vi "SectionA04_Week3_Stus.vi"() -> ()   [LabVIEW 2013]
uses:
  <vilib>/Platform/NI_3dgraph.lvlib
panel:
  in  "Bits":dbl(knob) scale=0.0..10.0
  in  "3D Surface":refnum<k7>(container)
  out "2^Bits":dbl
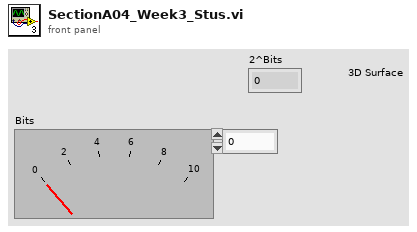
[diagram p1: front panel]
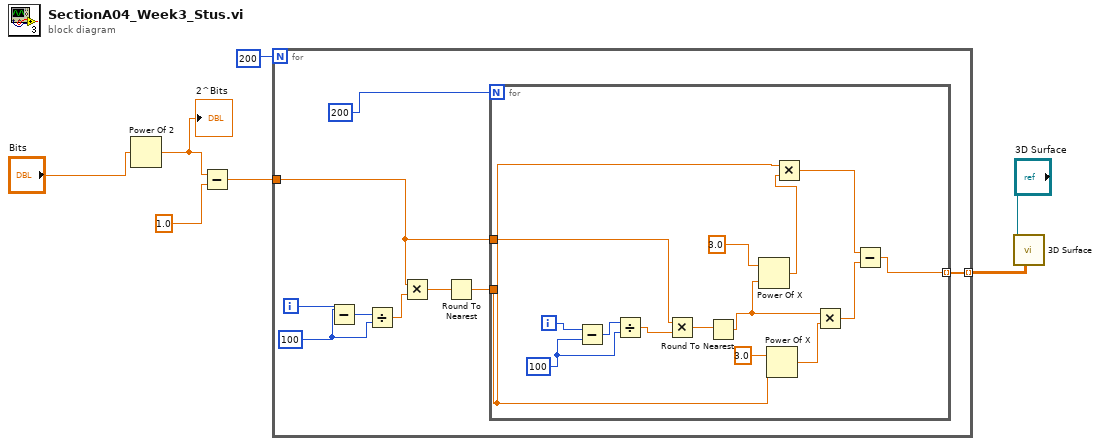
[diagram p0: block diagram]
diagram:
  n1 = Power Of 2(x="Bits") -> (2^x=w7:dbl)
  "2^Bits" <- w7
  n2 = Subtract(x=w7, y=1.0) -> (x-y=w5:dbl)
  n3 = for {
    N: 200 -> [_]
    tunnel: w5 -> [w10]
    tunnel: [w9] -> w2 mode=indexing
    i -> [w12]
    w8 = 100
    n4 = Subtract(x=w8, y=w12) -> (x-y=w16:i32)
    n5 = Divide(x=w16, y=w8) -> (x/y=w15:dbl)
    n6 = Multiply(x=w10, y=w15) -> (x*y=w14:dbl)
    n7 = Round To Nearest(number=w14) -> (nearest integer value=w11:dbl)
    n8 = for {
      N: 200 -> [_]
      tunnel: w11 -> [w20]
      tunnel: w10 -> [w26]
      tunnel: [w17] -> w9 mode=indexing
      i -> [w31]
      w28 = 100
      n9 = Subtract(x=w31, y=w28) -> (x-y=w29:i32)
      n10 = Divide(x=w29, y=w28) -> (x/y=w27:dbl)
      n11 = Multiply(x=w26, y=w27) -> (x*y=w30:dbl)
      n12 = Round To Nearest(number=w30) -> (nearest integer value=w25:dbl)
      n13 = Power Of X(1:w25, 2:3.0) -> (0:w21:dbl)
      n14 = Power Of X(1:w20, 2:3.0) -> (0:w24:dbl)
      n15 = Multiply(x=w20, y=w21) -> (x*y=w22:dbl)
      n16 = Multiply(x=w25, y=w24) -> (x*y=w23:dbl)
      n17 = Subtract(x=w22, y=w23) -> (x-y=w17:dbl)
    }
  }
  n18 = call <vilib>:"3D Surface.vi"("z matrix"=w2, "3D graph"="3D Surface") -> ()  [unwired: 8 in, 2 out]
